vi "Get Model Parameter File Path.vi"(8 "error in (no error)":errorcluster) -> (0 "error out":errorcluster, 3 "Model Parameter Path":path caption="selected path")   [LabVIEW 2016, in "System Mapping Tool.lvlib"]
uses:
  System Mapping Tool.lvlib
  <vilib>/Utility/config.llb/Read Key (Path).vi
  <vilib>/Utility/config.llb/Write Key (Path).vi
  <vilib>/Utility/config.llb/NI_LVConfig.lvlib
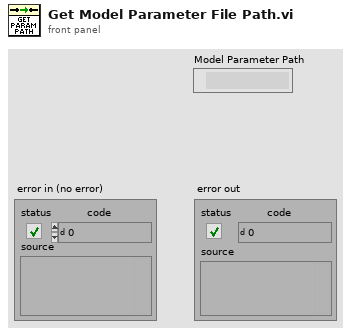
[diagram p1: front panel]
types:
  T1 = typedef "NI_LVConfig.lvlib/Config Data RefNum.ctl" = refnum<k1>
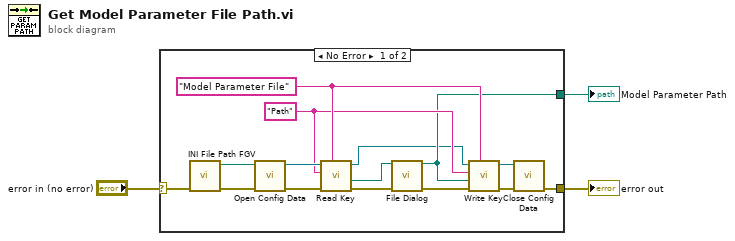
[diagram p0: block diagram]
diagram:
  n1 = case shown="No Error" "error in (no error)" {
    selector: "error in (no error)" -> [w18 w19]
    tunnel: [w9 _] -> w3
    tunnel: [w6 w19] -> w1
    frame No Error {
      w10 = "Path"
      w11 = "Model Parameter File"
      n2 = call "INI File Path FGV.vi"("error in (no error)"=w18) -> ("error out"=w17:errorcluster, "Path"=w15:path)  [unwired: 9 in]
      n3 = call <vilib>:"Open Config Data.vi"("error in (no error)"=w17, "configuration file path"=w15) -> ("error out"=w16:errorcluster, "refnum"=w14:T1)  [unwired: 7 in, 1 out]
      n4 = call-poly <vilib>:"Read Key.vi"("section"=w11, "error in (no error)"=w16, "key"=w10, "refnum"=w14) -> ("error out"=w13:errorcluster, "value"=w12:path, "refnum out"=w4:T1)  [unwired: 4 in, 1 out]
      n5 = call "File Dialog"("start path"=w12, "error in"=w13) -> ("selected path"=w9:path, "error out"=w5:errorcluster)  [unwired: 10 in, 2 out]
      n6 = call-poly <vilib>:"Write Key.vi"("section"=w11, "error in (no error)"=w5, "value"=w9, "key"=w10, "refnum"=w4) -> ("error out"=w8:errorcluster, "refnum out"=w7:T1)  [unwired: 4 in, 1 out]
      n7 = call <vilib>:"Close Config Data.vi"("error in (no error)"=w8, "refnum"=w7) -> ("error out"=w6:errorcluster)  [unwired: 8 in, 1 out]
    }
    frame Error {
    }
  }
  "Model Parameter Path" <- w3
  "error out" <- w1
